vi "Solo2RFID.vi"() -> ()   [LabVIEW 2019]
panel:
  out "Rfid 2":string
  in  "RFID VISA resource name 2":refnum<visa-resource-name>="COM18"
  out "Rfid":string
  in  "RFID VISA resource name":refnum<visa-resource-name>="COM5"
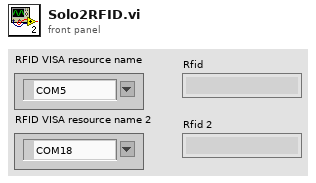
[diagram p1: front panel]
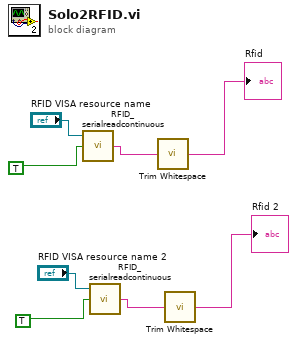
[diagram p0: block diagram]
diagram:
  n1 = call "RFID_serialreadcontinuous.vi"("Read 2"=TRUE, "VISA resource name"="RFID VISA resource name") -> ("Response 2"=w7:string)  [unwired: 1 in]
  n2 = call "RFID_serialreadcontinuous.vi"("Read 2"=TRUE, "VISA resource name"="RFID VISA resource name 2") -> ("Response 2"=w3:string)  [unwired: 1 in]
  n3 = call <vilib>:"Trim Whitespace.vi"("string"=w7) -> ("trimmed string"=→"Rfid":string)  [unwired: 1 in]
  n4 = call <vilib>:"Trim Whitespace.vi"("string"=w3) -> ("trimmed string"=→"Rfid 2":string)  [unwired: 1 in]
